vi "Quadratic Roots.vi"() -> ()   [LabVIEW 2025]
panel:
  out "Root 2":dbl
  out "Root 1":dbl
  in  "B":dbl
  in  "C":dbl
  in  "A":dbl
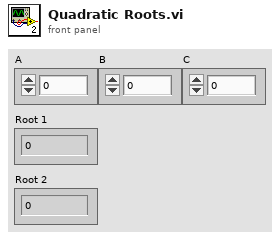
[diagram p1: front panel]
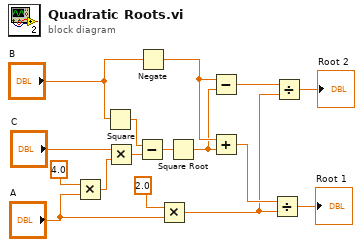
[diagram p0: block diagram]
diagram:
  n1 = Multiply(x=4.0, y="A") -> (x*y=w14:dbl)
  n2 = Square(x="B") -> (x^2=w12:dbl)
  n3 = Multiply(x="C", y=w14) -> (x*y=w11:dbl)
  n4 = Subtract(x=w12, y=w11) -> (x-y=w10:dbl)
  n5 = Negate(x="B") -> (-x=w5:dbl)
  n6 = Multiply(x=2.0, y="A") -> (x*y=w1:dbl)
  n7 = Square Root(x=w10) -> (sqrt(x)=w4:dbl)
  n8 = Subtract(x=w5, y=w4) -> (x-y=w2:dbl)
  n9 = Add(x=w5, y=w4) -> (x+y=w7:dbl)
  n10 = Divide(x=w7, y=w1) -> (x/y=→"Root 1":dbl)
  n11 = Divide(x=w2, y=w1) -> (x/y=→"Root 2":dbl)
